vi "Get Stop Button Status.vi"(8 "Error In":errorcluster) -> (0 "Error Out":errorcluster, 3 "Stop ButtonOut":bool)   [LabVIEW 2014]
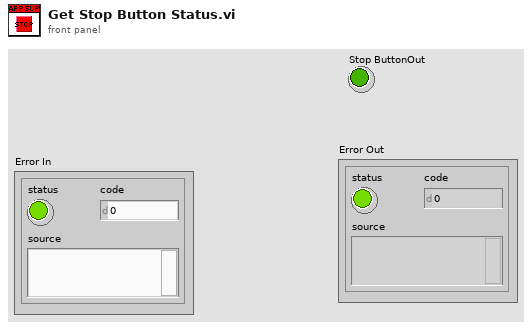
[diagram p1: front panel]
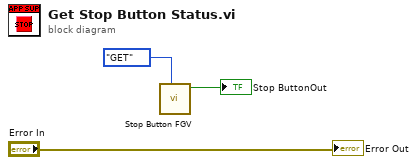
[diagram p0: block diagram]
diagram:
  n1 = call "Stop Button FGV.vi"("Operation"=enum16{"GET", "SET"}."GET") -> ("Stop ButtonOut"=→"Stop ButtonOut":bool)  [unwired: 10 in]
  "Error Out" <- "Error In"
